vi "GetSerialNum.vi"(6 "Enable":bool, 8 "error in (no error)":errorcluster, 10 "Cluster":T1, 11 "VISA Refnum in":refnum<visa-resource-name>) -> (0 "error out":errorcluster, 1 "Serial num":u16, 2 "Firmware":u16, 3 "VISA Refnum OUT":refnum<visa-resource-name>, 4 "p_atm":sgl)   [LabVIEW 2020]
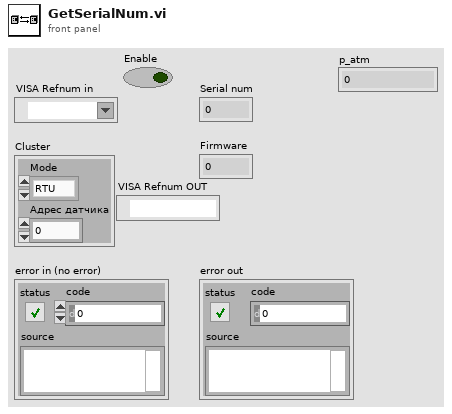
[diagram p1: front panel]
types:
  T1 = cluster{"Mode":enum16{"RTU", "ASCII"}, "Адрес датчика":u16}
  T2 = cluster{"Mode":enum16{"RTU", "ASCII"}, "Новый адрес датчика":u16}
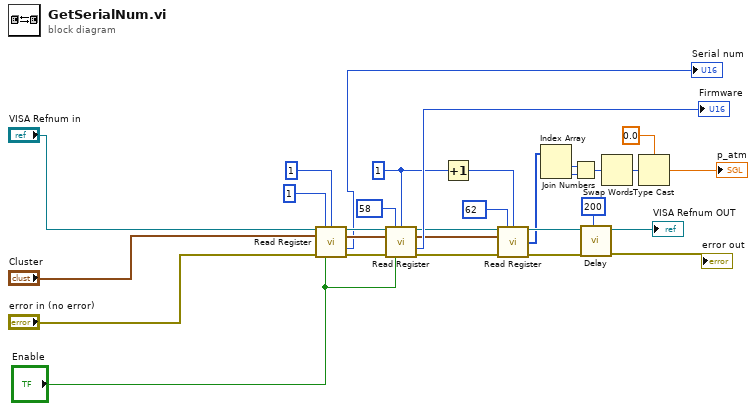
[diagram p0: block diagram]
diagram:
  w9 = u16 1 ("Holding Register")
  n1 = call "Read Register.vi"("Refnum in"="VISA Refnum in", "startReg"=u16 1 ("Holding Register"), "Quantity"=u16 1 ("Holding Register"), "Mode"="Cluster", "error in (no error)"="error in (no error)", "Enable"="Enable") -> ("Refnum Out"=w28:refnum<visa-resource-name>, "ModeOut"=w27:T2, "Numeric"=→"Serial num":u16, "error out"=w26:errorcluster)  [unwired: 5 in, 1 out]
  n2 = call "Read Register.vi"("Refnum in"=w28, "startReg"=u16 58 ("mask (16)"), "Quantity"=w9, "Mode"=w27, "error in (no error)"=w26, "Enable"="Enable") -> ("Refnum Out"=w16:refnum<visa-resource-name>, "ModeOut"=w12:T2, "Numeric"=→"Firmware":u16, "error out"=w14:errorcluster)  [unwired: 5 in, 1 out]
  n3 = Increment(x=w9) -> (x+1=w8:u16)
  n4 = call "Read Register.vi"("Refnum in"=w16, "startReg"=u16 62 ("mask (16)"), "Quantity"=w8, "Mode"=w12, "error in (no error)"=w14) -> ("Refnum Out"=w15:refnum<visa-resource-name>, "Holding Registers"=w3:u16[], "error out"=w13:errorcluster)  [unwired: 6 in, 2 out]
  n5 = Index Array(array=w3) -> (element #1=w6:u16, element #2=w7:u16)  [unwired: 2 in]
  n6 = Join Numbers(hi=w6, lo=w7) -> ((hi.lo)=w5:u32)
  n7 = call "Delay.vi"("milliseconds to wait"=u32 200, "error in (no error)"=w13, "VISA Refnum  In"=w15) -> ("error out"=→"error out":errorcluster, "VISA Refnum out"=→"VISA Refnum OUT":refnum<visa-resource-name>)  [unwired: 7 in]
  n8 = Swap Words(1:w5) -> (0:w4:u32)
  n9 = Type Cast(type=sgl 0.0 ("p_atm"), x=w4) -> (*(type *) &x=→"p_atm":sgl)
